vi "Write command.vi"(8 "error in":errorcluster, 10 "Command":string, 11 "VISA Refnum in":refnum<visa-resource-name>) -> (0 "error out":errorcluster, 2 "String":string, 3 "VISA Refnum out":refnum<visa-resource-name>)   [LabVIEW 2020, in "Arduino-Adafruit stepper.lvlib"]
uses:
  Arduino-Adafruit stepper.lvlib
  <vilib>/Instr/_visa.llb/VISA Flush IO Buffer Mask.ctl
  8c92989d-46b5-4006-83e4-ac9dabb44d55.vi
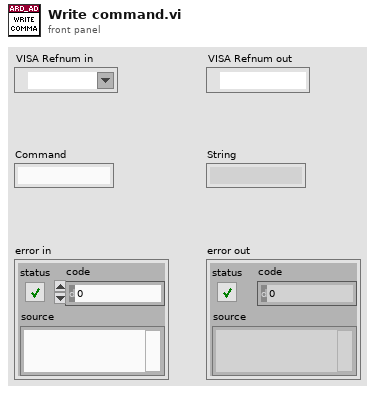
[diagram p1: front panel]
types:
  T1 = typedef "VISA Flush IO Buffer Mask.ctl" = u16
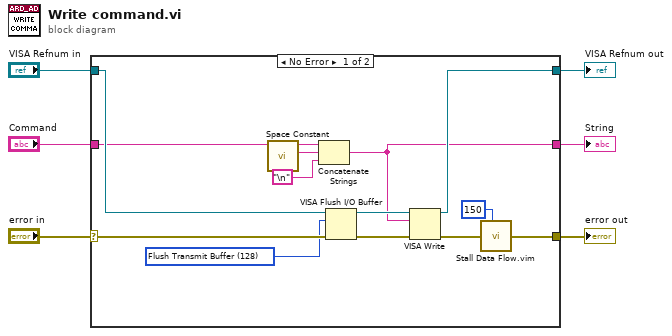
[diagram p0: block diagram]
diagram:
  n1 = case shown="No Error" "error in" {
    selector: "error in" -> [w17 w21]
    tunnel: "VISA Refnum in" -> [w16 w20]
    tunnel: [w19 w20] -> w3
    tunnel: [w8 w21] -> w1
    tunnel: "Command" -> [w12 _]
    tunnel: [w9 _] -> w2
    frame No Error {
      w13 = T1 128 items=["Flush Receive Buffer"=16, "Write Transmit Buffer to Device"=32, "Flush Receive Buffer (No I/O)"=64, "Flush Transmit Buffer"=128] ("Mask")
      n2 = call <vilib>:"Space Constant.vi"() -> ("String"=w11:string)
      n3 = Concatenate Strings(w12, w11, "\n") -> (w9:string)
      n4 = VISA Flush I/O Buffer(VISA resource name=w16, mask (16)=w13, error in (no error)=w17) -> (VISA resource name out=w15:refnum<visa-resource-name>, error out=w14:errorcluster)
      n5 = VISA Write(VISA resource name=w15, write buffer=w9, error in (no error)=w14) -> (VISA resource name out=w19:refnum<visa-resource-name>, error out=w18:errorcluster)  [unwired: 1 out]
      n6 = call "Stall Data Flow.vim"("value in"=w18, "milliseconds to wait"=u32 150) -> ("value out"=w8:errorcluster)  [unwired: 1 out]
    }
    frame Error {
    }
  }
  "VISA Refnum out" <- w3
  "String" <- w2
  "error out" <- w1
